vi "PPR-simulate-dashboard.vi"() -> ()   [LabVIEW 2019]
uses:
  <vilib>/Rock Robotics/WPI/ThirdParty/JAS_Junk/TrajLib/TypeDef/POSE2D.ctl
  <vilib>/Rock Robotics/WPI/ThirdParty/JAS_Junk/TrajLib/TypeDef/TRANSLATION2D.ctl
  <vilib>/Rock Robotics/WPI/ThirdParty/JAS_Junk/TrajLib/TypeDef/ROTATION2D.ctl
  <vilib>/Rock Robotics/WPI/ThirdParty/MJansen/PathPlanner/TypeDef/PathPlannerTrajectory.ctl
  <vilib>/Rock Robotics/WPI/ThirdParty/MJansen/PathPlanner/TypeDef/PathPlannerTrajectoryState.ctl
  <vilib>/Rock Robotics/WPI/ThirdParty/MJansen/PathPlanner/TypeDef/PathPlannerPathConstraints.ctl
  Diff_Drive_System/PPR_DRIVE_GLOBALS.vi
  Simulation/PPR_SIM_SIM_Globals.vi
  Trajectory Following/PPR_TRAJECTORY_GLOBALS.vi
  Vision_Interface/PPS_Vision_Globals.vi
  <vilib>/Rock Robotics/WPI/ThirdParty/MJansen/PathPlanner/PathPlanner24.lvlib
  <vilib>/Rock Robotics/WPI/ThirdParty/JAS_Junk/TrajLib/Trajectory_Library.lvlib
panel:
  in  "Tab Control":T1(tab)
  out "Battery Voltage":dbl(graph)
  out "Drive Speed":cluster{"Motor Dmd":dbl, "Motor Dmd":dbl}(graph)
  out "Drive Motor Demands":cluster{"Motor Dmd":dbl, "Motor Dmd":dbl}(graph)
  out "GyroReading_Degreees":dbl format="%15.3f"
  out "Encoder Distances":dbl[](array[numeric]) format="%17.2f"
  out "Encoder Velocities":dbl[](array[numeric]) format="%17.2f"
  out "Motor Demands":dbl[](array[numeric]) format="%17.2f"
  out "Battery Volts":dbl format="%16.2f"
  out "Diff Module Devices":T2(array[cluster])
  out "Wheel \nSpeed Dmd":dbl[](array[numeric]) format="%17.3f"
  out "Diff Drive Motor output":T3(graph)
  out "Diff Drive Speed M/S":T4(graph)
  out "Diff Drive Speed Error  M/S":T5(graph)
  out "Closed Loop Control":bool
  out "Orientation Angle Dmd_Rad":dbl format="%17.3f"
  out "GyroHeading_Radians":dbl format="%17.2f"
  out "Orientation Angle Error_Rad":dbl format="%17.3f"
  out "Orientation Correct CO":dbl format="%17.3f"
  out "Wheel Out":dbl[](array[numeric]) format="%17.3f"
  out "Wheel \nSpeed M/S":dbl[](array[numeric]) format="%17.3f"
  out "Wheel Speed Err":dbl[](array[numeric]) format="%17.3f"
  out "Limited Wheel \nSpeed Dmd":dbl[](array[numeric]) format="%17.3f"
  out "Traj Heading Err DEG":dbl format="%17.2f"
  out "Traj Pos Err Ft":dbl format="%17.2f"
  out "Traj Y Err Ft":dbl format="%17.2f"
  out "Traj X Err Ft":dbl format="%17.2f"
  out "Vision Pose":T6={"TRANSLATION"={"X"=0.0, "Y"=0.0}, "ROTATION"={"VALUE"=0.0, "COS"=1.0, "SIN"=0.0}} {"ROTATION"."SIN" format="%13.4f"; "ROTATION"."COS" format="%13.4f"; "ROTATION"."VALUE" format="%13.4f"; "TRANSLATION"."Y" format="%14.3f"; "TRANSLATION"."X" format="%14.3f"}
  out "Vision\nPose":bool
  out "Trajectory Status":T9(graph)
  out "Trajectory Execution \nClosed Loop":bool
  out "Trajectory Error":T10(graph)
  out "Traj_OnTarget":bool
  out "Traj Heading Dmd Deg":dbl format="%17.2f"
  out "Traj Final Heading Dmd Deg":dbl format="%17.2f"
  out "Traj Sample Time Sec":dbl format="%17.2f"
  out "Traj Rot Vel FF Rad/Sec":dbl format="%17.2f"
  out "Relative Trajectory Pose":T6={"TRANSLATION"={"X"=0.0, "Y"=0.0}, "ROTATION"={"VALUE"=0.0, "COS"=1.0, "SIN"=0.0}} {"ROTATION"."SIN" format="%13.4f"; "ROTATION"."COS" format="%13.4f"; "ROTATION"."VALUE" format="%13.4f"; "TRANSLATION"."Y" format="%14.3f"; "TRANSLATION"."X" format="%14.3f"}
  out "Absolute Odometry \nPose":T6={"TRANSLATION"={"X"=0.0, "Y"=0.0}, "ROTATION"={"VALUE"=0.0, "COS"=1.0, "SIN"=0.0}} {"ROTATION"."SIN" format="%13.4f"; "ROTATION"."COS" format="%13.4f"; "ROTATION"."VALUE" format="%13.4f"; "TRANSLATION"."Y" format="%14.3f"; "TRANSLATION"."X" format="%14.3f"}
  out "Other ABS Odometry\nPose":T6={"TRANSLATION"={"X"=0.0, "Y"=0.0}, "ROTATION"={"VALUE"=0.0, "COS"=1.0, "SIN"=0.0}} {"ROTATION"."SIN" format="%13.4f"; "ROTATION"."COS" format="%13.4f"; "ROTATION"."VALUE" format="%13.4f"; "TRANSLATION"."Y" format="%14.3f"; "TRANSLATION"."X" format="%14.3f"}
  out "Absolue Trajectory":cluster{dbl[], dbl[]}(graph)
  out "Absolute Trajectory":T11 {"States"."TargetHolonomicRotation"."SIN" format="%13.4f"; "States"."TargetHolonomicRotation"."COS" format="%13.4f"; "States"."TargetHolonomicRotation"."VALUE" format="%13.4f"; "States"."Heading"."SIN" format="%13.4f"; "States"."Heading"."COS" format="%13.4f"; "States"."Heading"."VALUE" format="%13.4f"; "States"."PositionMeters"."Y" format="%14.3f"; "States"."PositionMeters"."X" format="%14.3f"}
  out "Relative Trajectory":cluster{dbl[], dbl[]}(graph)
  # "SIMULATION"
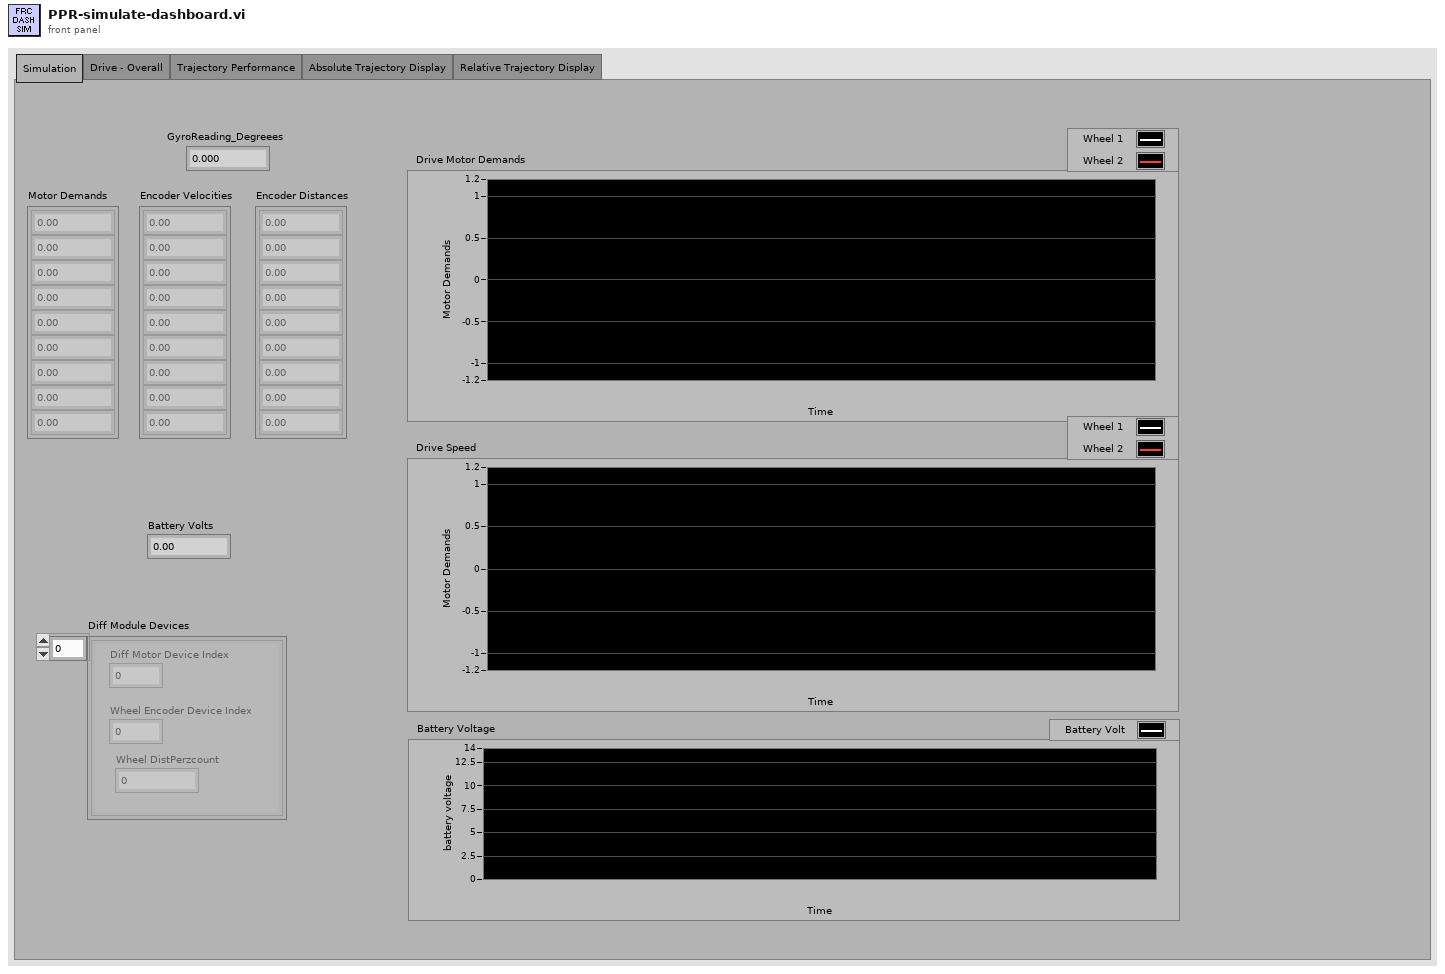
[diagram p1: front panel]
types:
  T1 = enum32{"Simulation", "Drive - Overall", "Trajectory Performance", "Absolute Trajectory Display", "Relative Trajectory Display"}
  T2 = cluster{"Diff Motor Device Index":i32, "Wheel Encoder Device Index":i32, "Wheel DistPerzcount":dbl}[]
  T3 = cluster{"Left Wheel Motor Out":dbl, "Right Wheel Motor Out":dbl}
  T4 = cluster{"Left Wheel Speed M/S":dbl, "Right Wheel Speed M/S":dbl}
  T5 = cluster{"Left Wheel Speed Err M/S":dbl, "Right Wheel Speed Err M/S":dbl}
  T6 = typedef "Trajectory_Library.lvlib/POSE2D.ctl" = cluster{"TRANSLATION":T7, "ROTATION":T8}
  T7 = typedef "Trajectory_Library.lvlib/TRANSLATION2D.ctl" = cluster{"X":dbl, "Y":dbl}
  T8 = typedef "Trajectory_Library.lvlib/ROTATION2D.ctl" = cluster{"VALUE":dbl, "COS":dbl, "SIN":dbl}
  T9 = cluster{dbl, dbl, dbl, "Traj_Sample_Time_Sec":dbl}
  T10 = cluster{"Traj X Err":dbl, "Traj Y Err":dbl, "Traj Heading Err":dbl}
  T11 = typedef "PathPlanner24.lvlib/PathPlannerTrajectory.ctl" = cluster{"States":T12[]}
  T12 = typedef "PathPlanner24.lvlib/PathPlannerTrajectoryState.ctl" = cluster{"TimeSeconds":dbl, "VelocityMPS":dbl, "AccerationMpsSq":dbl, "HeadingAngularVelRadPerSec":dbl, "PositionMeters":T7, "Heading":T8, "TargetHolonomicRotation":T8, "CurvatureRadPerMeter":dbl, "PathPlannerConstraints":T13, "DeltaPos":dbl}
  T13 = typedef "PathPlanner24.lvlib/PathPlannerPathConstraints.ctl" = cluster{"MaxVelocityMps;":dbl, "MaxAccelerationMpsSq;":dbl, "MaxAngularVelRadPsEc;":dbl, "MaxAngularAccRadPSecSq":dbl, "Exists":bool}
  T14 = cluster{"Traj X Err_FT":dbl, "Traj Y Err_FT":dbl, "Traj Heading Err_DEG":dbl}
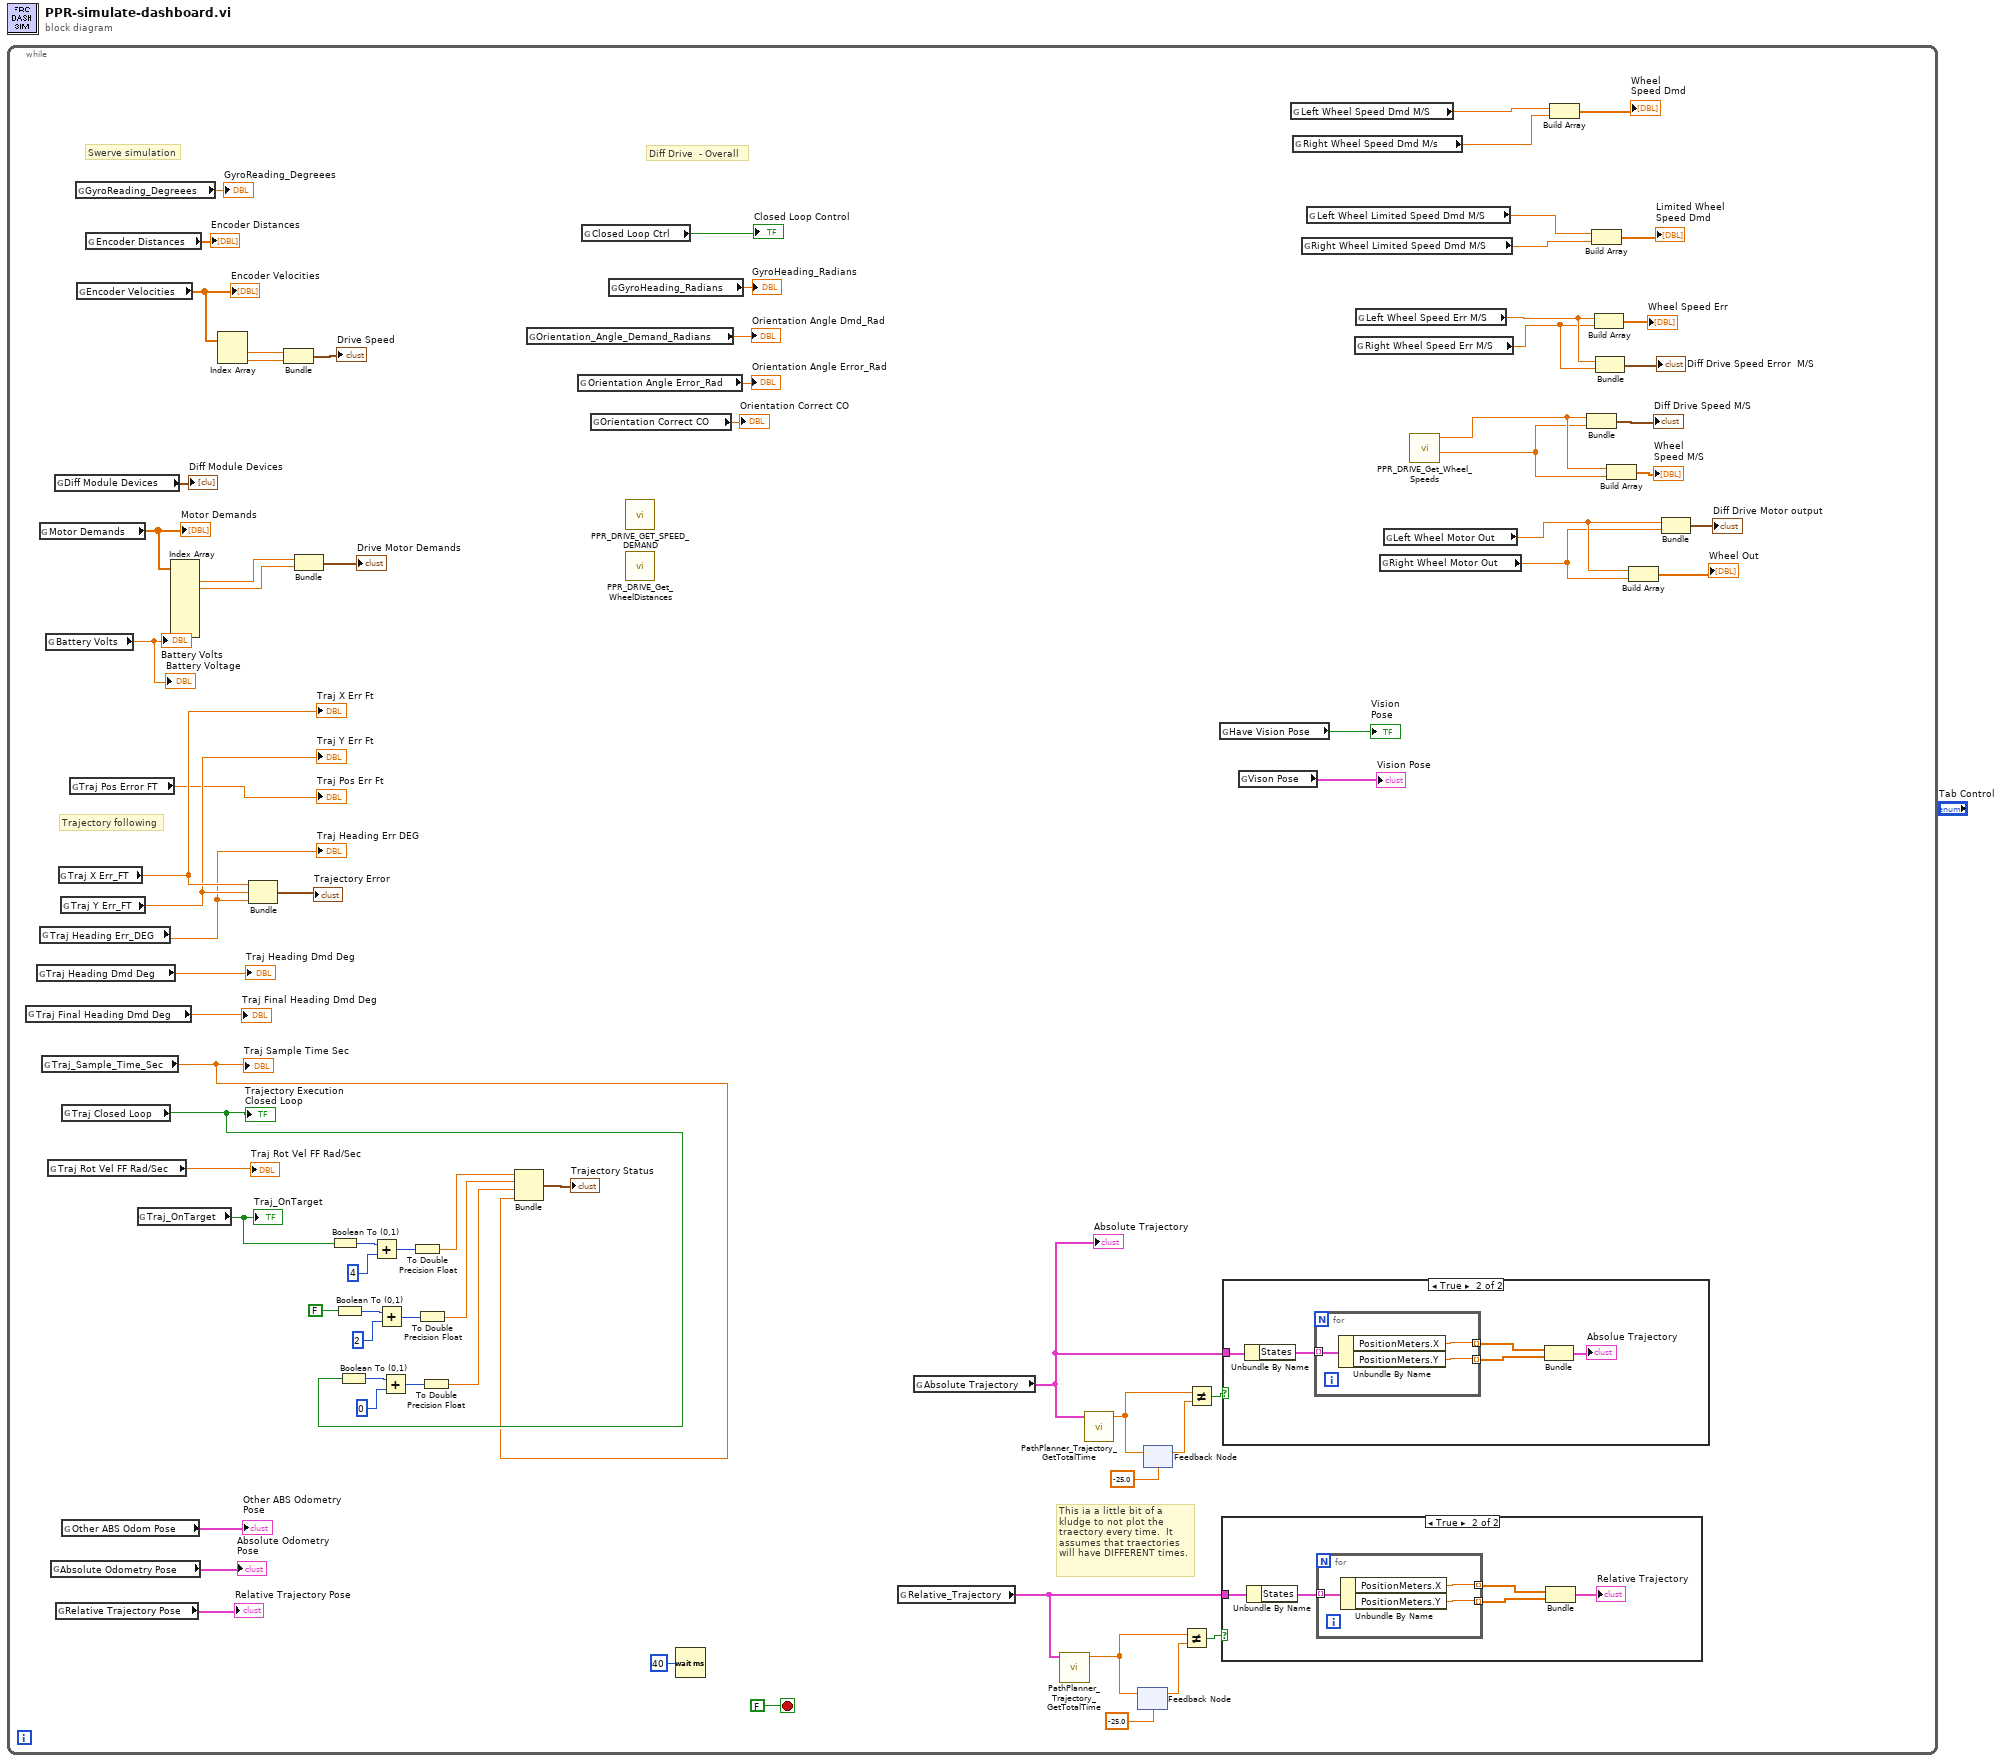
[diagram p0: block diagram]
diagram:
  n1 = while {
    stop <- FALSE stop-if-true
    # "This ia a little bit of a \nkludge to not plot the\ntraectory every time.  It \nassumes that traectories\nwill have DIFFERENT times."
    # "Trajectory following"
    # "Swerve simulation"
    # "Diff Drive  - Overall"
    n2 = global read "PPR_TRAJECTORY_GLOBALS.vi" "Traj Final Heading Dmd Deg"() -> (→"Traj Final Heading Dmd Deg":dbl)
    n3 = global read "PPR_TRAJECTORY_GLOBALS.vi" "Traj Heading Dmd Deg"() -> (→"Traj Heading Dmd Deg":dbl)
    n4 = global read "PPR_SIM_SIM_Globals.vi" "Motor Demands"() -> (w68:dbl[])
    "Motor Demands" <- w68
    n5 = global read "PPR_TRAJECTORY_GLOBALS.vi" "Traj Heading Err_DEG"() -> (w2:dbl)
    "Traj Heading Err DEG" <- w2
    n6 = global read "PPR_TRAJECTORY_GLOBALS.vi" "Traj_Sample_Time_Sec"() -> (w47:dbl)
    "Traj Sample Time Sec" <- w47
    n7 = global read "PPR_SIM_SIM_Globals.vi" "Battery Volts"() -> (→"Battery Volts" →"Battery Voltage":dbl)
    n8 = global read "PPR_TRAJECTORY_GLOBALS.vi" "Traj Rot Vel FF Rad/Sec"() -> (→"Traj Rot Vel FF Rad/Sec":dbl)
    n9 = global read "PPR_TRAJECTORY_GLOBALS.vi" "Absolute Odometry Pose"() -> (→"Absolute Odometry \nPose":T6)
    n10 = global read "PPR_SIM_SIM_Globals.vi" "Diff Module Devices"() -> (→"Diff Module Devices":T2)
    n11 = global read "PPR_TRAJECTORY_GLOBALS.vi" "Relative Trajectory Pose"() -> (→"Relative Trajectory Pose":T6)
    n12 = global read "PPR_TRAJECTORY_GLOBALS.vi" "Traj X Err_FT"() -> (w4:dbl)
    "Traj X Err Ft" <- w4
    n13 = global read "PPR_TRAJECTORY_GLOBALS.vi" "Traj Y Err_FT"() -> (w3:dbl)
    "Traj Y Err Ft" <- w3
    n14 = global read "PPR_TRAJECTORY_GLOBALS.vi" "Traj Closed Loop"() -> (w49:bool)
    "Trajectory Execution \nClosed Loop" <- w49
    n15 = global read "PPR_TRAJECTORY_GLOBALS.vi" "Other ABS Odom Pose"() -> (→"Other ABS Odometry\nPose":T6)
    n16 = global read "PPR_TRAJECTORY_GLOBALS.vi" "Traj Pos Error FT"() -> (→"Traj Pos Err Ft":dbl)
    n17 = global read "PPR_SIM_SIM_Globals.vi" "GyroReading_Degreees"() -> (→"GyroReading_Degreees":dbl)
    n18 = global read "PPR_SIM_SIM_Globals.vi" "Encoder Velocities"() -> (w8:dbl[])
    "Encoder Velocities" <- w8
    n19 = global read "PPR_SIM_SIM_Globals.vi" "Encoder Distances"() -> (→"Encoder Distances":dbl[])
    n20 = global read "PPR_TRAJECTORY_GLOBALS.vi" "Traj_OnTarget"() -> (w61:bool)
    "Traj_OnTarget" <- w61
    n21 = Index Array(array=w68) -> (element #1=w67:dbl, element #2=w9:dbl)  [unwired: 8 in, 6 out]
    n22 = Index Array(array=w8) -> (element #1=w7:dbl, element #2=w6:dbl)  [unwired: 2 in]
    n23 = Bundle("Traj X Err_FT"=w4, "Traj Y Err_FT"=w3, "Traj Heading Err_DEG"=w2) -> (→"Trajectory Error":T14)  [unwired: 1 in]
    n24 = Bundle("Motor Dmd"=w7, "Motor Dmd"=w6) -> (→"Drive Speed":cluster{"Motor Dmd":dbl, "Motor Dmd":dbl})  [unwired: 1 in]
    n25 = Bundle("Motor Dmd"=w67, "Motor Dmd"=w9) -> (→"Drive Motor Demands":cluster{"Motor Dmd":dbl, "Motor Dmd":dbl})  [unwired: 1 in]
    n26 = Boolean To (0,1)(Boolean=w61) -> (0, 1=w59:i16)
    n27 = Boolean To (0,1)(Boolean=FALSE) -> (0, 1=w56:i16)
    n28 = Boolean To (0,1)(Boolean=w49) -> (0, 1=w52:i16)
    n29 = Add(x=w59, y=i16 4) -> (x+y=w58:i16)
    n30 = Add(x=w56, y=i16 2) -> (x+y=w55:i16)
    n31 = Add(x=w52, y=i16 0) -> (x+y=w51:i16)
    n32 = To Double Precision Float(number=w58) -> (double precision float=w60:dbl)
    n33 = To Double Precision Float(number=w55) -> (double precision float=w53:dbl)
    n34 = To Double Precision Float(number=w51) -> (double precision float=w48:dbl)
    n35 = Bundle(w60, w53, w48, "Traj_Sample_Time_Sec"=w47) -> (→"Trajectory Status":T9)  [unwired: 1 in]
    n36 = global read "PPR_DRIVE_GLOBALS.vi" "Orientation_Angle_Demand_Radians"() -> (→"Orientation Angle Dmd_Rad":dbl)
    n37 = global read "PPR_DRIVE_GLOBALS.vi" "Orientation Angle Error_Rad"() -> (→"Orientation Angle Error_Rad":dbl)
    n38 = global read "PPR_DRIVE_GLOBALS.vi" "Closed Loop Ctrl"() -> (→"Closed Loop Control":bool)
    n39 = global read "PPR_DRIVE_GLOBALS.vi" "Orientation Correct CO"() -> (→"Orientation Correct CO":dbl)
    n40 = global read "PPR_DRIVE_GLOBALS.vi" "GyroHeading_Radians"() -> (→"GyroHeading_Radians":dbl)
    n41 = call "PPR_DRIVE_GET_SPEED_DEMAND.vi"() -> ()  [unwired: 10 in, 2 out]
    n42 = call "PPR_DRIVE_Get_WheelDistances.vi"() -> ()  [unwired: 10 in, 2 out]
    n43 = Wait (ms)(milliseconds to wait=u32 40) -> ()  [unwired: 1 out]
    n44 = global read "PPR_TRAJECTORY_GLOBALS.vi" "Relative_Trajectory"() -> (w29:T11)
    n45 = global read "PPR_TRAJECTORY_GLOBALS.vi" "Absolute Trajectory"() -> (w31:T11)
    "Absolute Trajectory" <- w31
    n46 = call <vilib>:"PathPlanner_Trajectory_GetTotalTime.vi"("PathPlannerTrajectory"=w29) -> ("TotalTimeSeconds"=w28:dbl)  [unwired: 10 in]
    n47 = call <vilib>:"PathPlanner_Trajectory_GetTotalTime.vi"("PathPlannerTrajectory"=w31) -> ("TotalTimeSeconds"=w30:dbl)  [unwired: 10 in]
    n48 = feedback #1(-25.0 ("TotalTime_Sec")) -> (w33:dbl)
    n49 = feedback-in #1(w28) -> ()
    n50 = feedback #2(-25.0 ("TotalTime_Sec")) -> (w36:dbl)
    n51 = feedback-in #2(w30) -> ()
    n52 = Not Equal?(x=w28, y=w33) -> (x != y?=w32:bool)
    n53 = Not Equal?(x=w30, y=w36) -> (x != y?=w35:bool)
    n54 = global read "PPS_Vision_Globals.vi" "Have Vision Pose"() -> (→"Vision\nPose":bool)
    n55 = case shown="True" w32 {
      tunnel: w29 -> [_ w79]
      frame False {
      }
      frame True {
        n56 = Unbundle By Name(w79) -> ("States"=w80:T12[])
        n57 = for {
          tunnel: [w85] -> w81 mode=indexing
          tunnel: [w84] -> w82 mode=indexing
          tunnel: w80 -> [w83] mode=indexing
          n58 = Unbundle By Name(w83) -> ("PositionMeters.X"=w85:dbl, "PositionMeters.Y"=w84:dbl)
        }
        n59 = Bundle(w81, w82) -> (→"Relative Trajectory":cluster{dbl[], dbl[]})  [unwired: 1 in]
      }
    }
    n60 = case shown="True" w35 {
      tunnel: w31 -> [_ w86]
      frame False {
      }
      frame True {
        n61 = Unbundle By Name(w86) -> ("States"=w88:T12[])
        n62 = for {
          tunnel: [w93] -> w89 mode=indexing
          tunnel: [w92] -> w90 mode=indexing
          tunnel: w88 -> [w91] mode=indexing
          n63 = Unbundle By Name(w91) -> ("PositionMeters.X"=w93:dbl, "PositionMeters.Y"=w92:dbl)
        }
        n64 = Bundle(w89, w90) -> (→"Absolue Trajectory":cluster{dbl[], dbl[]})  [unwired: 1 in]
      }
    }
    n65 = global read "PPS_Vision_Globals.vi" "Vison Pose"() -> (→"Vision Pose":T6)
    n66 = global read "PPR_DRIVE_GLOBALS.vi" "Left Wheel Speed Dmd M/S"() -> (w14:dbl)
    n67 = global read "PPR_DRIVE_GLOBALS.vi" "Right Wheel Speed Dmd M/s"() -> (w13:dbl)
    n68 = global read "PPR_DRIVE_GLOBALS.vi" "Right Wheel Limited Speed Dmd M/S"() -> (w10:dbl)
    n69 = global read "PPR_DRIVE_GLOBALS.vi" "Left Wheel Limited Speed Dmd M/S"() -> (w11:dbl)
    n70 = global read "PPR_DRIVE_GLOBALS.vi" "Right Wheel Speed Err M/S"() -> (w16:dbl)
    n71 = global read "PPR_DRIVE_GLOBALS.vi" "Left Wheel Speed Err M/S"() -> (w17:dbl)
    n72 = global read "PPR_DRIVE_GLOBALS.vi" "Right Wheel Motor Out"() -> (w22:dbl)
    n73 = global read "PPR_DRIVE_GLOBALS.vi" "Left Wheel Motor Out"() -> (w23:dbl)
    n74 = call "PPR_DRIVE_Get_Wheel_Speeds.vi"() -> ("Right Wheel Speed M/S"=w19:dbl, "Left Wheel Speed M/S"=w20:dbl)  [unwired: 10 in]
    n75 = Build Array(w14, w13) -> (→"Wheel \nSpeed Dmd":dbl[])
    n76 = Bundle("Left Wheel Speed M/S"=w20, "Right Wheel Speed M/S"=w19) -> (→"Diff Drive Speed M/S":T4)  [unwired: 1 in]
    n77 = Build Array(w11, w10) -> (→"Limited Wheel \nSpeed Dmd":dbl[])
    n78 = Build Array(w17, w16) -> (→"Wheel Speed Err":dbl[])
    n79 = Bundle("Left Wheel Speed Err M/S"=w17, "Right Wheel Speed Err M/S"=w16) -> (→"Diff Drive Speed Error  M/S":T5)  [unwired: 1 in]
    n80 = Build Array(w20, w19) -> (→"Wheel \nSpeed M/S":dbl[])
    n81 = Build Array(w23, w22) -> (→"Wheel Out":dbl[])
    n82 = Bundle("Left Wheel Motor Out"=w23, "Right Wheel Motor Out"=w22) -> (→"Diff Drive Motor output":T3)  [unwired: 1 in]
  }
